vi "uManagerRearrangeStr.vi"(0 "numImg":u32, 5 "AcqSettingsIn":string, 7 "labViewComIn":string, 9 "start":dbl, 12 "expTime":dbl) -> (4 "AcqSettingsOut":string, 6 "labViewComOut":string)   [LabVIEW 2021]
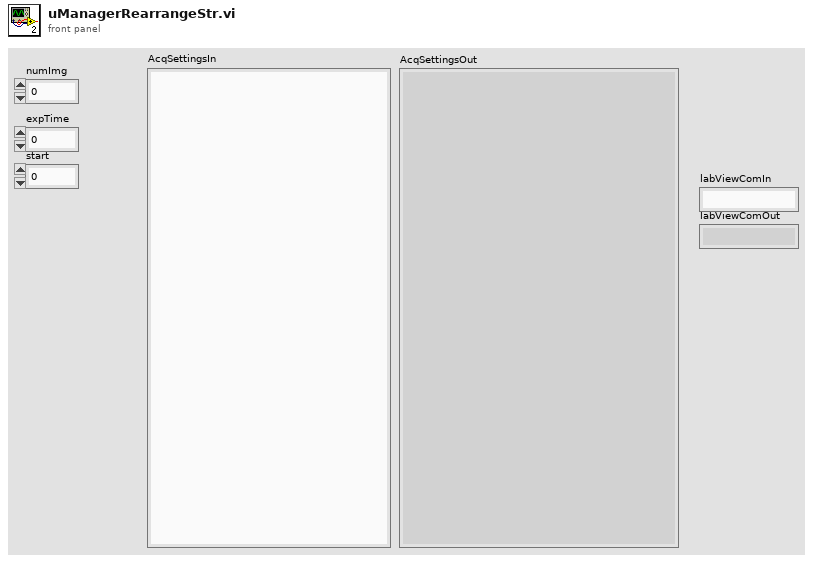
[diagram p1: front panel]
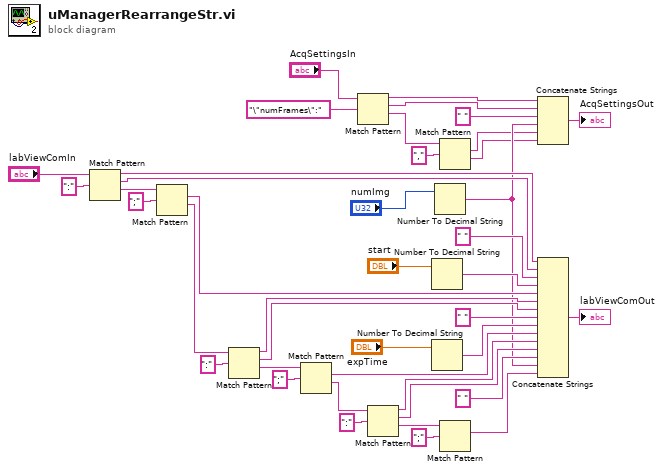
[diagram p0: block diagram]
diagram:
  n1 = Match Pattern(string="labViewComIn", regular expression=":") -> (before substring=w29:string, match substring=w28:string, after substring=w39:string)  [unwired: 1 in, 1 out]
  n2 = Match Pattern(string=w39, regular expression=";") -> (match substring=w15:string, after substring=w27:string)  [unwired: 1 in, 2 out]
  n3 = Match Pattern(string=w27, regular expression=":") -> (before substring=w24:string, match substring=w23:string, after substring=w36:string)  [unwired: 1 in, 1 out]
  n4 = Match Pattern(string=w36, regular expression=";") -> (match substring=w12:string, after substring=w30:string)  [unwired: 1 in, 2 out]
  n5 = Match Pattern(string="AcqSettingsIn", regular expression="\"numFrames\":") -> (before substring=w7:string, match substring=w6:string, after substring=w11:string)  [unwired: 1 in, 1 out]
  n6 = Match Pattern(string=w30, regular expression=":") -> (before substring=w20:string, match substring=w19:string, after substring=w33:string)  [unwired: 1 in, 1 out]
  n7 = Number To Decimal String(number="start") -> (decimal integer string=w14:string)  [unwired: 1 in]
  n8 = Number To Decimal String(number="expTime") -> (decimal integer string=w13:string)  [unwired: 1 in]
  n9 = Number To Decimal String(number="numImg") -> (decimal integer string=w5:string)  [unwired: 1 in]
  n10 = Match Pattern(string=w11, regular expression=",") -> (match substring=w3:string, after substring=w2:string)  [unwired: 1 in, 2 out]
  n11 = Match Pattern(string=w33, regular expression=";") -> (match substring=w16:string)  [unwired: 1 in, 3 out]
  n12 = Concatenate Strings(w7, w6, " " ("string"), w5, w3, w2) -> (→"AcqSettingsOut":string)
  n13 = Concatenate Strings(w29, w28, " " ("string"), w14, w15, w24, w23, " " ("string"), w13, w12, w20, w19, " " ("string"), w5, w16) -> (→"labViewComOut":string)
